vi "批次号.vi"(11 "批次码":string caption="字符串") -> ()   [LabVIEW 2020]
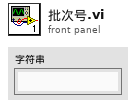
[diagram p1: front panel]
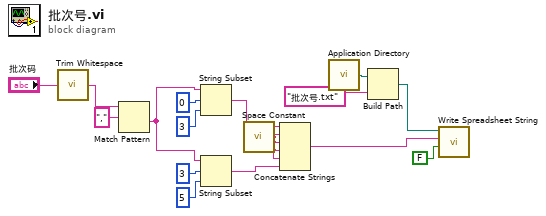
[diagram p0: block diagram]
diagram:
  n1 = call <vilib>:"Trim Whitespace.vi"("string"="批次码") -> ("trimmed string"=w3:string)  [unwired: 1 in]
  n2 = Match Pattern(string=w3, regular expression="," ("正则表达式")) -> (after substring=w1:string)  [unwired: 1 in, 3 out]
  n3 = String Subset(string=w1, offset (0)=0 ("偏移量(0)"), length (rest)=3 ("长度（剩余）")) -> (substring=w7:string)
  n4 = String Subset(string=w1, offset (0)=3 ("偏移量(0)"), length (rest)=5 ("长度（剩余）")) -> (substring=w5:string)
  n5 = call <vilib>:"Space Constant.vi"() -> ("String"=w6:string)
  n6 = Concatenate Strings(w7, w6, w6, w6, w6, w5) -> (w4:string)
  n7 = call <vilib>:"Application Directory.vi"() -> ("Application Directory"=w12:path)
  n8 = Build Path(base path=w12, name or relative path="批次号.txt" ("名称或相对路径")) -> (appended path=w10:path)
  n9 = call <vilib>:"Write Spreadsheet String.vi"("append to file? (new file:F)"=FALSE, "spreadsheet string"=w4, "file path (dialog if empty)"=w10) -> ()  [unwired: 7 in, 2 out]
